vi "RegisterSubscriber.vi"(1 "ROS":T1) -> (0 "XML":string)   [LabVIEW 2010]
uses:
  SubVIs/_ROSControl.ctl
  SubVIs/_ROSDirection.ctl
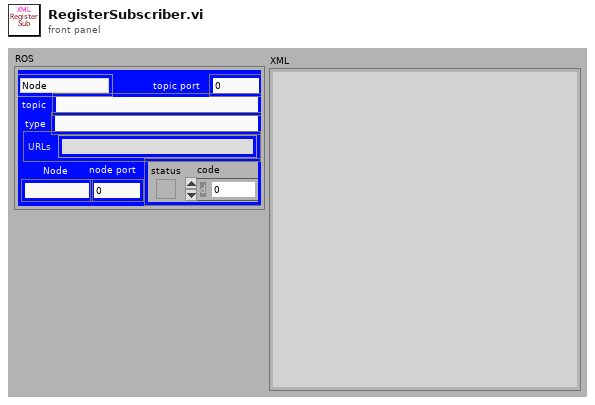
[diagram p1: front panel]
types:
  T1 = typedef "_ROSControl.ctl" = cluster{"topic port":u16, "Node":string, "topic":string, "type":string, "node port":u32, "error ":errorcluster, "Direction":T2, "APIs":string[]}
  T2 = typedef "_ROSDirection.ctl" = enum16{"Node", "Publisher", "Subscriber", "Service Client"}
  T3 = enum16{"http://IP:port", "http://IP", "IP:port", "IP only"}
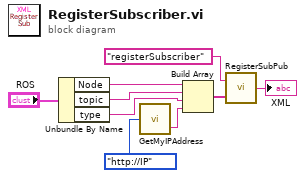
[diagram p0: block diagram]
diagram:
  n1 = Unbundle By Name("ROS") -> ("Node"=w6:string, "topic"=w7:string, "type"=w8:string)
  n2 = call "GetMyIPAddress.vi"("Format"=T3."http://IP") -> ("URI"=w9:string)  [unwired: 3 in]
  n3 = Build Array(w6, w7, w8, w9) -> (w3:string[])
  n4 = call "RegisterSubPub.vi"("Parameters"=w3, "MethodName"="registerSubscriber") -> ("XML"=→"XML":string)
